vi "VisionTest1.vi"() -> ()   [LabVIEW 2019]
uses:
  <vilib>/Analysis/coordinate.llb/2D Cartesian Coordinate Shift (Array).vi
  <vilib>/Analysis/coordinate.llb/2D Cartesian Coordinate Rotation (Array).vi
  <vilib>/vision/NI_Vision_Development_Module.lvlib
  <vilib>/Analysis/NI_AALPro.lvlib
  KNRm_ReMi_OS6_436Motor.lvlibp
panel:
  out "error in (no error) 2":errorcluster
  out "y":dbl
  out "x":dbl
  out "stop":bool
  out "botton":bool
  in  "y":dbl=8.0 format="%#_13g"
  out "ColorDet Img":T1(plugin-control)
  out "G":u16
  out "B":u16
  out "Class":string
  out "output Brick (x, y, theta)":dbl[](array[numeric])
  in  "Grab":bool
  in  "Range (Threshold 1)":cluster{"Lower value":sgl, "Upper value":sgl}={"Lower value"=61.0, "Upper value"=255.0}
  out "Particle Measurements (Real-World) (Particle Analysis 1)":dbl[][](array[numeric]) format="%.2f"
  in  "BCG Values (Brightness 1)":T2={"Brightness"=100.0, "Contrast"=50.0, "Gamma"=0.5}
  out "Number of Matches (Pattern Matching 1)":i32
  out "Cal Img":T1(plugin-control)
  out "Bin Img":T1(plugin-control)
  in  "Stop Button":bool
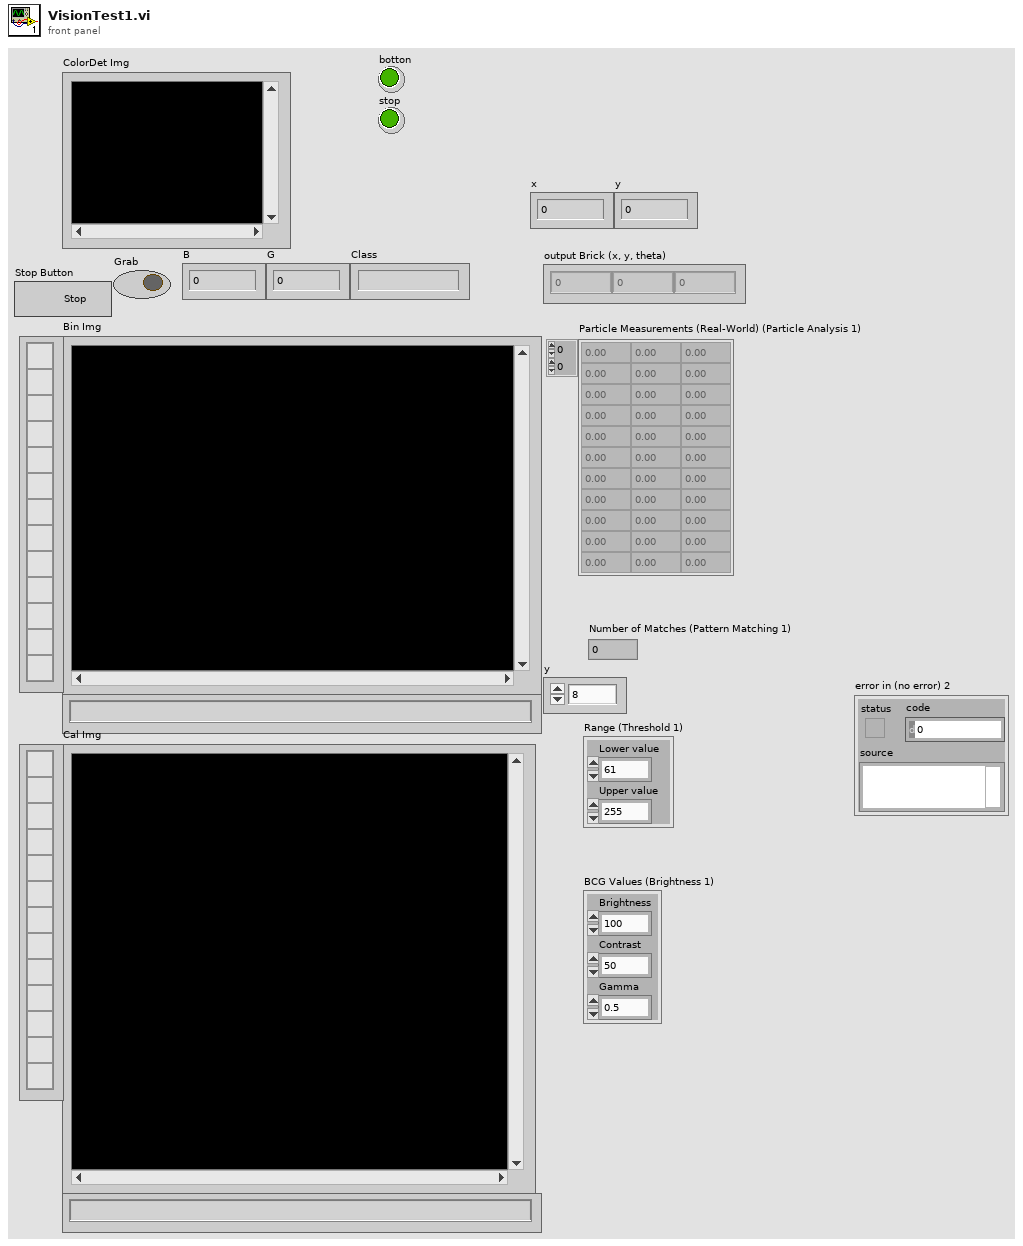
[diagram p1: front panel]
types:
  T1 = typedef "IMAQ Image.ctl" = refnum<image>
  T2 = cluster{"Brightness":sgl, "Contrast":sgl, "Gamma":sgl}
  T3 = typedef "Image Type" = u32
  T4 = cluster{"Numeric":u8, "Numeric":u8, "Numeric":u8, "Numeric":u8}
  T5 = cluster{"Interpolation Type":enum32{"Zero Order", "Bilinear", "Quadratic", "Cubic", "Bilinear Fixed"}, "Destination Width":u32, "Destination Height":u32, "Fill Value":sgl}
  T6 = cluster{"Particle Measurements (Real-World) (Particle Analysis 1)":dbl[], "Class":string}
  T7 = enum16{"P1", "P2", "P3", "P4", "P5", "P6", "OUT", "take a picture"}
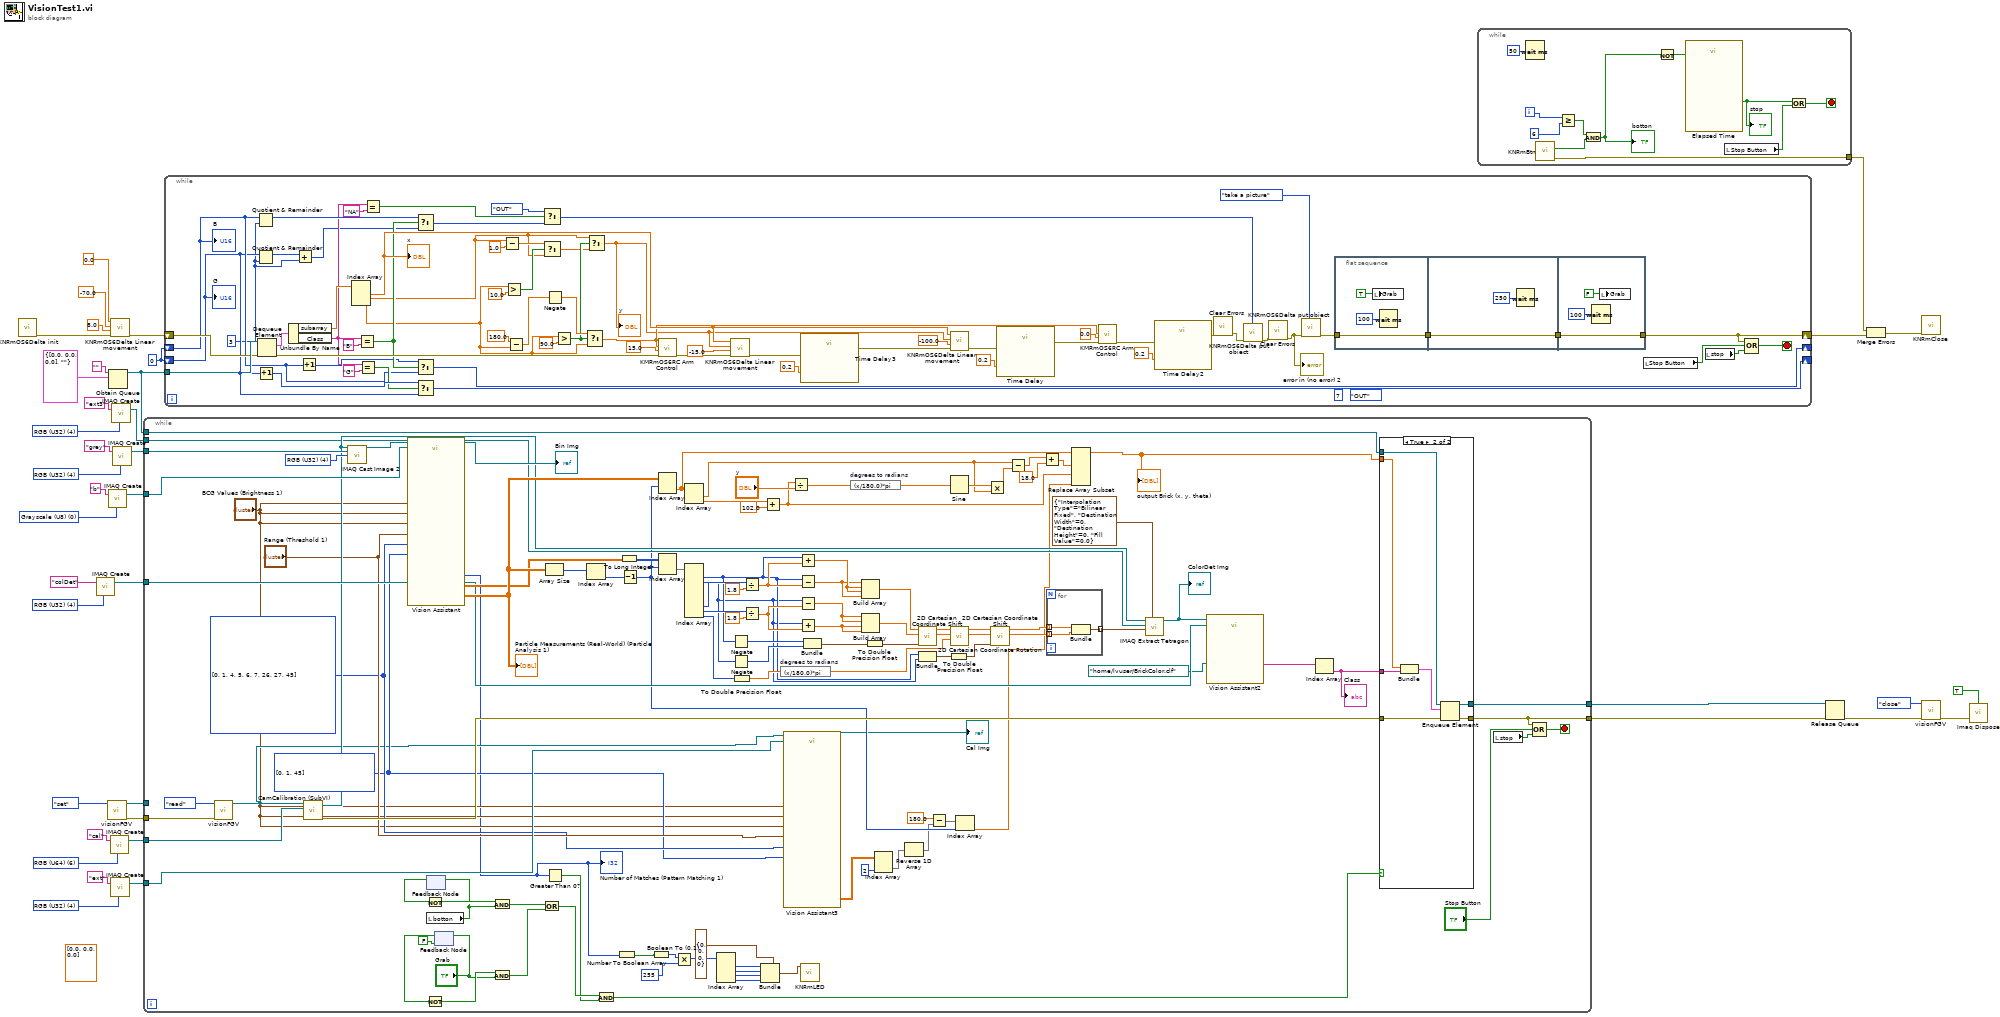
[diagram p0: block diagram]
diagram:
  w5 = T3 4 items=["Grayscale (U8)", "Grayscale (I16)", "Grayscale (SGL)", "Complex (CSG)", "RGB (U32)", "HSL (U32)", "RGB (U64)", "Grayscale (U16)"] ("Image Type")
  w7 = u16 0
  w10 = T3 4 items=["Grayscale (U8)", "Grayscale (I16)", "Grayscale (SGL)", "Complex (CSG)", "RGB (U32)", "HSL (U32)", "RGB (U64)", "Grayscale (U16)"] ("Image Type")
  (unwired) dbl[] [0.0, 0.0, 0.0] ("subarray")
  w24 = T3 0 items=["Grayscale (U8)", "Grayscale (I16)", "Grayscale (SGL)", "Complex (CSG)", "RGB (U32)", "HSL (U32)", "RGB (U64)", "Grayscale (U16)"] ("Image Type")
  w27 = T3 4 items=["Grayscale (U8)", "Grayscale (I16)", "Grayscale (SGL)", "Complex (CSG)", "RGB (U32)", "HSL (U32)", "RGB (U64)", "Grayscale (U16)"] ("Image Type")
  w30 = T3 6 items=["Grayscale (U8)", "Grayscale (I16)", "Grayscale (SGL)", "Complex (CSG)", "RGB (U32)", "HSL (U32)", "RGB (U64)", "Grayscale (U16)"] ("Image Type")
  w32 = T3 4 items=["Grayscale (U8)", "Grayscale (I16)", "Grayscale (SGL)", "Complex (CSG)", "RGB (U32)", "HSL (U32)", "RGB (U64)", "Grayscale (U16)"] ("Image Type")
  n1 = call "KNRmOS6Delta init.vi"() -> ("error out"=w18:errorcluster)  [unwired: 11 in]
  n2 = call "IMAQ Create"("Image Name"="colDet", "Image Type"=w10) -> ("New Image"=w9:T1)  [unwired: 3 in, 1 out]
  n3 = call "visionFGV.vi"("Function"=enum16{"set", "read", "close"}."set") -> ("error out"=w34:errorcluster, "Image Out fgv"=w38:T1)  [unwired: 9 in]
  n4 = call "IMAQ Create"("Image Name"="b", "Image Type"=w24) -> ("New Image"=w22:T1)  [unwired: 3 in, 1 out]
  n5 = Obtain Queue(name (unnamed)="", element data type=cluster{"subarray":dbl[], "Class":string} {"subarray"=[0.0, 0.0, 0.0], "Class"=""}) -> (queue out=w16:refnum<queue>)  [unwired: 3 in, 2 out]
  n6 = call "IMAQ Create"("Image Name"="cal", "Image Type"=w30) -> ("New Image"=w28:T1)  [unwired: 3 in, 1 out]
  n7 = call "KNRmOS6Delta Linear movement.vi"("error in (no error)"=w18, "z0"=8.0, "y0"=-70.0, "x0"=0.0) -> ("error out"=w15:errorcluster)  [unwired: 7 in]
  n8 = call "IMAQ Create"("Image Name"="ext", "Image Type"=w27) -> ("New Image"=w26:T1)  [unwired: 3 in, 1 out]
  n9 = call "IMAQ Create"("Image Name"="ext3", "Image Type"=w5) -> ("New Image"=w4:T1)  [unwired: 3 in, 1 out]
  n10 = call "IMAQ Create"("Image Name"="grey", "Image Type"=w32) -> ("New Image"=w31:T1)  [unwired: 3 in, 1 out]
  n11 = while {
    tunnel: w38 -> [_]
    tunnel: w34 -> [w148]
    tunnel: w31 -> [w147]
    tunnel: w28 -> [w146]
    tunnel: w26 -> [w65]
    tunnel: w22 -> [w144]
    tunnel: w16 -> [w143]
    tunnel: [w85] -> w14
    tunnel: [w141] -> w12
    tunnel: w9 -> [w128]
    tunnel: w4 -> [w124]
    stop <- w82 stop-if-true
    w63 = i32[] [0, 1, 4, 5, 6, 7, 26, 27, 45] items=["Center of Mass X", "Center of Mass Y", "First Pixel X", "First Pixel Y", "Bounding Rect Left", "Bounding Rect Top", "Bounding Rect Right", "Bounding Rect Bottom", "Max Feret Diameter Start X", "Max Feret Diameter Start Y", "Max Feret Diameter End X", "Max Feret Diameter End Y", "Max Horiz. Segment Length Left", "Max Horiz. Segment Length Right", "Max Horiz. Segment Length Row", "-", "Bounding Rect Width", "Bounding Rect Height", "Bounding Rect Diagonal", "Perimeter", "Convex Hull Perimeter", "Holes' Perimeter", "Max Feret Diameter", "Equivalent Ellipse Major Axis", "Equivalent Ellipse Minor Axis", "Equivalent Ellipse Minor Axis (Feret)", "Equivalent Rect Long Side", "Equivalent Rect Short Side", "Equivalent Rect Diagonal", "Equivalent Rect Short Side (Feret)", "Average Horiz. Segment Length", "Average Vert. Segment Length", "Hydraulic Radius", "Waddel Disk Diameter", "-", "Area", "Holes' Area", "Particle & Holes' Area", "Convex Hull Area", "Image Area", "-", "Number of Holes", "Number of Horiz. Segments", "Number of Vert. Segments", "-", "Orientation", "Max Feret Diameter Orientation", "-", "% Area/Image Area", "% Area/(Particle & Holes' Area)", "Ratio of Equivalent Ellipse Axes", "Ratio of Equivalent Rect Sides", "-", "Elongation Factor", "Compactness Factor", "Heywood Circularity Factor", "Type Factor", "-", "Sum X", "Sum Y", "Sum XX", "Sum XY", "Sum YY", "Sum XXX", "Sum XXY", "Sum XYY", "Sum YYY", "-", "Moment of Inertia XX", "Moment of Inertia XY", "Moment of Inertia YY", "Moment of Inertia XXX", "Moment of Inertia XXY", "Moment of Inertia XYY", "Moment of Inertia YYY", "Norm. Moment of Inertia XX", "Norm. Moment of Inertia XY", "Norm. Moment of Inertia YY", "Norm. Moment of Inertia XXX", "Norm. Moment of Inertia XXY", "Norm. Moment of Inertia XYY", "Norm. Moment of Inertia YYY", "Hu Moment 1", "Hu Moment 2", "Hu Moment 3", "Hu Moment 4", "Hu Moment 5", "Hu Moment 6", "Hu Moment 7"] ("Pixel Measurements (Particle Analysis 1)")
    w62 = i32[] [0, 1, 45] items=["Center of Mass X", "Center of Mass Y", "First Pixel X", "First Pixel Y", "Bounding Rect Left", "Bounding Rect Top", "Bounding Rect Right", "Bounding Rect Bottom", "Max Feret Diameter Start X", "Max Feret Diameter Start Y", "Max Feret Diameter End X", "Max Feret Diameter End Y", "Max Horiz. Segment Length Left", "Max Horiz. Segment Length Right", "Max Horiz. Segment Length Row", "-", "Bounding Rect Width", "Bounding Rect Height", "Bounding Rect Diagonal", "Perimeter", "Convex Hull Perimeter", "Holes' Perimeter", "Max Feret Diameter", "Equivalent Ellipse Major Axis", "Equivalent Ellipse Minor Axis", "Equivalent Ellipse Minor Axis (Feret)", "Equivalent Rect Long Side", "Equivalent Rect Short Side", "Equivalent Rect Diagonal", "Equivalent Rect Short Side (Feret)", "Average Horiz. Segment Length", "Average Vert. Segment Length", "Hydraulic Radius", "Waddel Disk Diameter", "-", "Area", "Holes' Area", "Particle & Holes' Area", "Convex Hull Area", "Image Area", "-", "Number of Holes", "Number of Horiz. Segments", "Number of Vert. Segments", "-", "Orientation", "Max Feret Diameter Orientation", "-", "% Area/Image Area", "% Area/(Particle & Holes' Area)", "Ratio of Equivalent Ellipse Axes", "Ratio of Equivalent Rect Sides", "-", "Elongation Factor", "Compactness Factor", "Heywood Circularity Factor", "Type Factor", "-", "Sum X", "Sum Y", "Sum XX", "Sum XY", "Sum YY", "Sum XXX", "Sum XXY", "Sum XYY", "Sum YYY", "-", "Moment of Inertia XX", "Moment of Inertia XY", "Moment of Inertia YY", "Moment of Inertia XXX", "Moment of Inertia XXY", "Moment of Inertia XYY", "Moment of Inertia YYY", "Norm. Moment of Inertia XX", "Norm. Moment of Inertia XY", "Norm. Moment of Inertia YY", "Norm. Moment of Inertia XXX", "Norm. Moment of Inertia XXY", "Norm. Moment of Inertia XYY", "Norm. Moment of Inertia YYY", "Hu Moment 1", "Hu Moment 2", "Hu Moment 3", "Hu Moment 4", "Hu Moment 5", "Hu Moment 6", "Hu Moment 7"] ("Real-World Measurements (Particle Analysis 1)")
    w149 = T3 4 items=["Grayscale (U8)", "Grayscale (I16)", "Grayscale (SGL)", "Complex (CSG)", "RGB (U32)", "HSL (U32)", "RGB (U64)", "Grayscale (U16)"] ("Image Type")
    n12 = call "visionFGV.vi"("Error In"=w148, "Function"=enum16{"set", "read", "close"}."read") -> ("Image Out fgv"=w61:T1)  [unwired: 8 in, 1 out]
    n13 = call "CamCalibration (SubVI).vi"("Image Dst"=w146, "Image In"=w61) -> ("error out"=w142:errorcluster, "Image Out"=w126:T1)  [unwired: 8 in]
    n14 = call "IMAQ Cast Image 2"("Image Src"=w126, "Image Dst"=w147, "Image Type"=w149) -> ("Image Dst Out"=w75:T1)  [unwired: 11 in, 1 out]
    n15 = call "Vision Assistant"("Image In"=w75, "Image Dst"=w144, "Red BCG Values (Brightness 1)"="BCG Values (Brightness 1)", "Range (Threshold 1)"="Range (Threshold 1)", "Pixel Measurements (Particle Analysis 1)"=w63, "Real-World Measurements (Particle Analysis 1)"=w62, "Green BCG Values (Brightness 1)"="BCG Values (Brightness 1)", "Blue BCG Values (Brightness 1)"="BCG Values (Brightness 1)") -> ("Image Out"=→"Bin Img":T1, "Number of Particles (Particle Analysis 1)"=w50:i32, "Particle Measurements (Real-World) (Particle Analysis 1)"=w136:dbl[][], "Particle Measurements (Pixels) (Particle Analysis 1)"=w130:dbl[][])  [unwired: 14 in, 2 out]
    "Number of Matches (Pattern Matching 1)" <- w50
    "Particle Measurements (Real-World) (Particle Analysis 1)" <- w136
    n16 = feedback #1() -> (w80:bool)  [unwired: 1 in]
    n17 = Not(x=w80) -> (.not. x?=w79:bool)
    n18 = local read "botton"() -> (w78:bool)
    n19 = feedback-in #1(w78) -> ()
    n20 = feedback-in #2("Grab") -> ()
    n21 = feedback #2(FALSE ("Grab")) -> (w140:bool)
    n22 = Not(x=w140) -> (.not. x?=w139:bool)
    n23 = And(x=w79, y=w78) -> (x .and. y?=w77:bool)
    n24 = And(x=w139, y="Grab") -> (x .and. y?=w89:bool)
    n25 = Or(x=w77, y=w89) -> (x .or. y?=w88:bool)
    n26 = Array Size(array=w136) -> (size(s)=w137:i32[])
    n27 = Greater Than 0?(x=w50) -> (x > 0?=w87:bool)
    n28 = Index Array(array=w137) -> (element=w135:i32)  [unwired: 1 in]
    n29 = And(x=w88, y=w87) -> (x .and. y?=w86:bool)
    n30 = Number To Boolean Array(number=w50) -> (Boolean array=w47:bool[])
    n31 = To Long Integer(number=w130) -> (32bit integer=w129:i32[][])
    n32 = Decrement(x=w135) -> (x-1=w66:i32)
    n33 = Boolean To (0,1)(Boolean=w47) -> (0, 1=w46:i16[])
    n34 = Index Array(array=w136, index (row)=w66) -> (element=w74:dbl[])  [unwired: 1 in]
    n35 = Index Array(array=w129, index (row)=w66) -> (element=w131:i32[])  [unwired: 1 in]
    n36 = Multiply(x=w46, y=255) -> (x*y=w45:i32[])
    n37 = Index Array(array=w74) -> (element #1=w67:dbl, element #2=w72:dbl)  [unwired: 2 in]
    n38 = Index Array(array=w131) -> (element #1=w106:i32, element #2=w105:i32, element #7=w116:i32, element #8=w112:i32, element #9=w119:i32)  [unwired: 9 in, 4 out]
    n39 = Index Array(array=w45) -> (element #1=w43:i32, element #2=w42:i32, element #3=w41:i32, element #4=w40:i32)  [unwired: 4 in]
    n40 = Negate(x=w106) -> (-x=w108:i32)
    n41 = Negate(x=w105) -> (-x=w109:i32)
    n42 = To Double Precision Float(number=w119) -> (double precision float=w110:dbl)
    n43 = Divide(x=w116, y=1.8) -> (x/y=w114:dbl)
    n44 = Divide(x=w112, y=1.8) -> (x/y=w111:dbl)
    n45 = Bundle(cluster=T4 {"Numeric"=0, "Numeric"=0, "Numeric"=0, "Numeric"=0} ("LEDSet"), "Numeric"=w43, "Numeric"=w42, "Numeric"=w41, "Numeric"=w40) -> (w48:T4)
    n46 = Add(x=w72, y=102.0) -> (x+y=w71:dbl)
    n47 = expression code="(x/180.0)*pi" "degrees to radians"(w110) -> (w118:dbl)
    n48 = call "Vision Assistant3"("Image In"=w61, "Image Dst"=w65, "Red BCG Values (Brightness 1)"="BCG Values (Brightness 1)", "Range (Threshold 1)"="Range (Threshold 1)", "Pixel Measurements (Particle Analysis 1)"=w63, "Real-World Measurements (Particle Analysis 1)"=w62, "Green BCG Values (Brightness 1)"="BCG Values (Brightness 1)", "Blue BCG Values (Brightness 1)"="BCG Values (Brightness 1)") -> ("Image Out"=→"Cal Img":T1, "Particle Measurements (Real-World) (Particle Analysis 1)"=w58:dbl[][])  [unwired: 14 in, 4 out]
    n49 = Divide(x=w71, y="y") -> (x/y=w133:dbl)
    n50 = Add(x=w106, y=w114) -> (x+y=w123:dbl)
    n51 = Subtract(x=w106, y=w114) -> (x-y=w122:dbl)
    n52 = Subtract(x=w105, y=w111) -> (x-y=w121:dbl)
    n53 = Add(x=w105, y=w111) -> (x+y=w120:dbl)
    n54 = call "KNRmLED.vi"("LEDSet"=w48) -> ()  [unwired: 10 in, 1 out]
    n55 = Bundle(w108, w109) -> (w107:cluster{i32, i32})  [unwired: 1 in]
    n56 = expression code="(x/180.0)*pi" "degrees to radians"(w133) -> (w94:dbl)
    n57 = Build Array(w122, w123, w123, w122) -> (w104:dbl[])
    n58 = Build Array(w121, w121, w120, w120) -> (w103:dbl[])
    n59 = To Double Precision Float(number=w107) -> (double precision float=w92:cluster{dbl, dbl})
    n60 = Index Array(array=w58, index (col)=2 ("disabled index (col)")) -> (element=w54:dbl[])  [unwired: 1 in]
    n61 = Reverse 1D Array(array=w54) -> (reversed array=w53:dbl[])
    n62 = call-poly <vilib>:"2D Cartesian Coordinate Shift.vi"("shift"=w92, "Y"=w103, "X"=w104) -> ("Y Out"=w101:dbl[], "X Out"=w102:dbl[])  [unwired: 6 in, 1 out]
    n63 = Bundle("Numeric"=w106, "Numeric"=w105) -> (w98:cluster{"Numeric":i32, "Numeric":i32})  [unwired: 1 in]
    n64 = Subtract(x=180.0, y=w53) -> (x-y=w55:dbl[])
    n65 = Sine(x=w94) -> (sin(x)=w91:dbl)
    n66 = call-poly <vilib>:"2D Cartesian Coordinate Rotation.vi"("theta"=w118, "Y"=w101, "X"=w102) -> ("Y Out"=w99:dbl[], "X Out"=w100:dbl[])  [unwired: 6 in, 1 out]
    n67 = To Double Precision Float(number=w98) -> (double precision float=w93:cluster{"Numeric":dbl, "Numeric":dbl})
    n68 = Index Array(array=w55, index=w66) -> (element=w52:dbl)
    n69 = Multiply(x=w91, y=w67) -> (x*y=w132:dbl)
    n70 = call-poly <vilib>:"2D Cartesian Coordinate Shift.vi"("shift"=w93, "Y"=w99, "X"=w100) -> ("Y Out"=w96:dbl[], "X Out"=w97:dbl[])  [unwired: 6 in, 1 out]
    n71 = Subtract(x=w67, y=w132) -> (x-y=w51:dbl)
    n72 = Add(x=w51, y=18.0) -> (x+y=w68:dbl)
    n73 = for {
      tunnel: w97 -> [w153] mode=indexing
      tunnel: w96 -> [w152] mode=indexing
      tunnel: [w151] -> w117 mode=indexing
      n74 = Bundle("Numeric"=w153, "Numeric"=w152) -> (w151:cluster{"Numeric":dbl, "Numeric":dbl})  [unwired: 1 in]
    }
    n75 = Replace Array Subset(array=w74, new element #1=w68, new element #2=w71, new element #3=w52) -> (w73:dbl[])  [unwired: 3 in]
    "output Brick (x, y, theta)" <- w73
    n76 = call-poly "IMAQ Extract Tetragon"("Options"=T5 {"Interpolation Type"=enum."Bilinear Fixed", "Destination Width"=0, "Destination Height"=0, "Fill Value"=0.0}, "Tetragon"=w117, "Image Dst"=w124, "Image Src"=w126) -> ("Image Dst Out"=w95:T1)  [unwired: 6 in, 1 out]
    "ColorDet Img" <- w95
    n77 = call "Vision Assistant2"("Image In"=w95, "Image Dst"=w128, "File Path (Color Classification 1)"=path "/home/lvuser/BrickColor.clf") -> ("Classes (Color Classification 1)"=w127:string[])  [unwired: 22 in, 2 out]
    n78 = Index Array(array=w127) -> (element=w90:string)  [unwired: 1 in]
    "Class" <- w90
    n79 = case shown="True" w86 {
      tunnel: w143 -> [w154 w162]
      tunnel: w73 -> [_ w158]
      tunnel: [w155 w161] -> w85
      tunnel: w142 -> [w155 w160]
      tunnel: [w154 w159] -> w141
      tunnel: w90 -> [_ w157]
      frame False {
      }
      frame True {
        n80 = Bundle("Particle Measurements (Real-World) (Particle Analysis 1)"=w158, "Class"=w157) -> (w156:T6)  [unwired: 1 in]
        n81 = Enqueue Element(queue=w162, element=w156, error in (no error)=w160) -> (queue out=w159:refnum<queue>, error out=w161:errorcluster)  [unwired: 1 in, 1 out]
      }
    }
    n82 = local read "stop"() -> (w83:bool)
    n83 = Compound Arithmetic op=OR(w85, "Stop Button", w83) -> (w82:bool)
  }
  n84 = while {
    tunnel: w16 -> [w227]
    shift-right: [w169] -> w2
    shift-left: w15 -> [w220]
    shift-right: [w193] -> _
    shift-left: w7 -> [w192]
    shift-right: [w194] -> _
    shift-left: w7 -> [w191]
    stop <- w174 stop-if-true
    w189 = u16 3 ("y")
    (unwired) T7."OUT" ("move to")
    (unwired) 7 ("y")
    n85 = Quotient & Remainder(x=w192, y=w189) -> (x-y*floor(x/y)=w199:u16)  [unwired: 1 out]
    n86 = Quotient & Remainder(x=w191, y=w189) -> (x-y*floor(x/y)=w190:u16)  [unwired: 1 out]
    n87 = Increment(x=w191) -> (x+1=w198:u16)
    n88 = Dequeue Element(queue=w227, error in (no error)=w220) -> (element=w207:cluster{"subarray":dbl[], "Class":string}, error out=w223:errorcluster)  [unwired: 1 in, 2 out]
    n89 = Unbundle By Name(w207) -> ("subarray"=w206:dbl[], "Class"=w196:string)
    n90 = Add(x=w190, y=w189) -> (x+y=w188:u16)
    n91 = Increment(x=w192) -> (x+1=w200:u16)
    n92 = Index Array(array=w206) -> (element #1=w215:dbl, element #2=w178:dbl, element #3=w177:dbl)  [unwired: 3 in]
    "x" <- w215
    n93 = Equal?(x=w196, y="B") -> (x = y?=w201:bool)
    n94 = Equal?(x=w196, y="G") -> (x = y?=w195:bool)
    n95 = Equal?(x=w196, y="NA") -> (x = y?=w204:bool)
    n96 = Select(t=w199, s=w201, f=w188) -> (s? t:f=w187:u16)
    n97 = Select(t=w200, s=w201, f=w192) -> (s? t:f=w193:u16)
    n98 = Select(t=w198, s=w195, f=w191) -> (s? t:f=w194:u16)
    n99 = Subtract(x=w178, y=1.0 ("y 2")) -> (x-y=w180:dbl)
    n100 = Greater?(x=w177, y=10.0) -> (0:w181:bool)
    n101 = Subtract(x=180.0, y=w177) -> (x-y=w209:dbl)
    n102 = Select(t=T7."OUT" ("move to"), s=w204, f=w187) -> (s? t:f=w186:u16)
    n103 = Select(t=w180, s=w181, f=w178) -> (s? t:f=w179:dbl)
    n104 = Negate(x=w209) -> (-x=w208:dbl)
    n105 = Greater?(x=w177, y=90.0) -> (0:w185:bool)
    n106 = Select(t=w208, s=w185, f=w177) -> (s? t:f=w210:dbl)
    n107 = Select(t=w178, s=w185, f=w179) -> (s? t:f=w183:dbl)
    "y" <- w183
    n108 = call "KMRmOS6RC Arm Control.vi"("error in (no error)"=w223, "clip"=15.0, "turn"=w210) -> ("error out"=w224:errorcluster)  [unwired: 6 in, 2 out]
    n109 = call "KNRmOS6Delta Linear movement.vi"("error in (no error)"=w224, "z0"=-15.0, "y0"=w183, "x0"=w215) -> ("error out"=w173:errorcluster)  [unwired: 7 in]
    n110 = call "Time Delay3"("error in (no error)"=w173, "Delay Time (s)"=0.2) -> ("error out"=w171:errorcluster)  [unwired: 9 in]
    n111 = call "KNRmOS6Delta Linear movement.vi"("error in (no error)"=w171, "z0"=-100.0, "y0"=w183, "x0"=w215) -> ("error out"=w216:errorcluster)  [unwired: 7 in]
    n112 = call "Time Delay"("error in (no error)"=w216, "Delay Time (s)"=0.2) -> ("error out"=w218:errorcluster)  [unwired: 9 in]
    n113 = call "KMRmOS6RC Arm Control.vi"("error in (no error)"=w218, "clip"=0.0, "turn"=w210) -> ("error out"=w214:errorcluster)  [unwired: 6 in, 2 out]
    n114 = call "Time Delay2"("error in (no error)"=w214, "Delay Time (s)"=0.2) -> ("error out"=w166:errorcluster)  [unwired: 9 in]
    n115 = call <vilib>:"Clear Errors.vi"("error in (no error)"=w166) -> ("error out"=w165:errorcluster)  [unwired: 5 in, 1 out]
    n116 = call "KNRmOS6Delta put obiect.vi"("move to"=w186, "error in (no error)"=w165) -> ("error in (no error) 2"=w164:errorcluster)  [unwired: 9 in]
    n117 = call <vilib>:"Clear Errors.vi"("error in (no error)"=w164) -> ("error out"=w163:errorcluster)  [unwired: 5 in, 1 out]
    "error in (no error) 2" <- w163
    n118 = call "KNRmOS6Delta put obiect.vi"("move to"=T7."take a picture", "error in (no error)"=w163) -> ("error in (no error) 2"=w170:errorcluster)  [unwired: 9 in]
    n119 = flat-sequence {
      tunnel: w170 -> [w230]
      tunnel: [w230] -> w167
      tunnel: [w231] -> w168
      tunnel: w167 -> [w231]
      tunnel: [w234] -> w169
      tunnel: w168 -> [w234]
      frame #0 {
        n120 = local write "Grab"(TRUE ("Grab")) -> ()
        n121 = Wait (ms)(milliseconds to wait=u32 100) -> ()  [unwired: 1 out]
      }
      frame #1 {
        n122 = Wait (ms)(milliseconds to wait=u32 250) -> ()  [unwired: 1 out]
      }
      frame #2 {
        n123 = Wait (ms)(milliseconds to wait=u32 100) -> ()  [unwired: 1 out]
        n124 = local write "Grab"(FALSE ("Grab")) -> ()
      }
    }
    n125 = local read "Stop Button"() -> (w176:bool)
    n126 = local read "stop"() -> (w175:bool)
    n127 = Compound Arithmetic op=OR(w169, w176, w175) -> (w174:bool)
    "B" <- w192
    "G" <- w191
  }
  n128 = while {
    tunnel: [w241] -> w3
    i -> [w240]
    stop <- w244 stop-if-true
    n129 = Wait (ms)(milliseconds to wait=u32 50) -> ()  [unwired: 1 out]
    n130 = call "KNRmBtn.vi"() -> ("error out"=w241:errorcluster, "myRIOButton"=w239:bool)  [unwired: 10 in]
    n131 = Greater Or Equal?(x=w240, y=6) -> (x >= y?=w237:bool)
    n132 = And(x=w237, y=w239) -> (x .and. y?=w238:bool)
    "botton" <- w238
    n133 = Not(x=w238) -> (.not. x?=w243:bool)
    n134 = call "Elapsed Time"("Reset"=w243) -> ("Time has Elapsed"=w246:bool)  [unwired: 11 in, 7 out]
    "stop" <- w246
    n135 = local read "Stop Button"() -> (w245:bool)
    n136 = Or(x=w246, y=w245) -> (x .or. y?=w244:bool)
  }
  n137 = Release Queue(queue=w12, error in (no error)=w14) -> (error out=w13:errorcluster)  [unwired: 1 in, 2 out]
  n138 = Merge Errors(w3, w2) -> (w1:errorcluster)
  n139 = call "KNRmClose.vi"("error in"=w1) -> ()  [unwired: 10 in, 1 out]
  n140 = call "visionFGV.vi"("Error In"=w13, "Function"=enum16{"set", "read", "close"}."close") -> ("error out"=w35:errorcluster)  [unwired: 8 in, 1 out]
  n141 = call "Imaq Dispose"("All Images? (No)"=TRUE, "error in (no error)"=w35) -> ()  [unwired: 4 in, 1 out]
